vi "Sub_Saveas.vi"(7 "Template Name":string="saveas.xlsx", 8 "row":i32=2, 10 "File Name":refnum<vi>, 11 "Path":refnum<vi>) -> (3 "Save Path":path)   [LabVIEW 2015]
uses:
  buffer_mode.ctl
  <vilib>/Utility/NIReport.llb/NI_report.lvclass
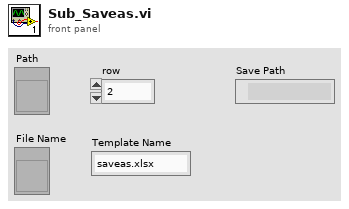
[diagram p1: front panel]
types:
  T1 = enum16{"maximized", "minimized", "normal", "no change"}
  T2 = enum16{"Standard Report", "HTML", "Word", "Excel"}
  T3 = typedef "buffer_mode.ctl" = enum16{"Clear", "Init", "Add 2nd data", "Delete", "Output"}
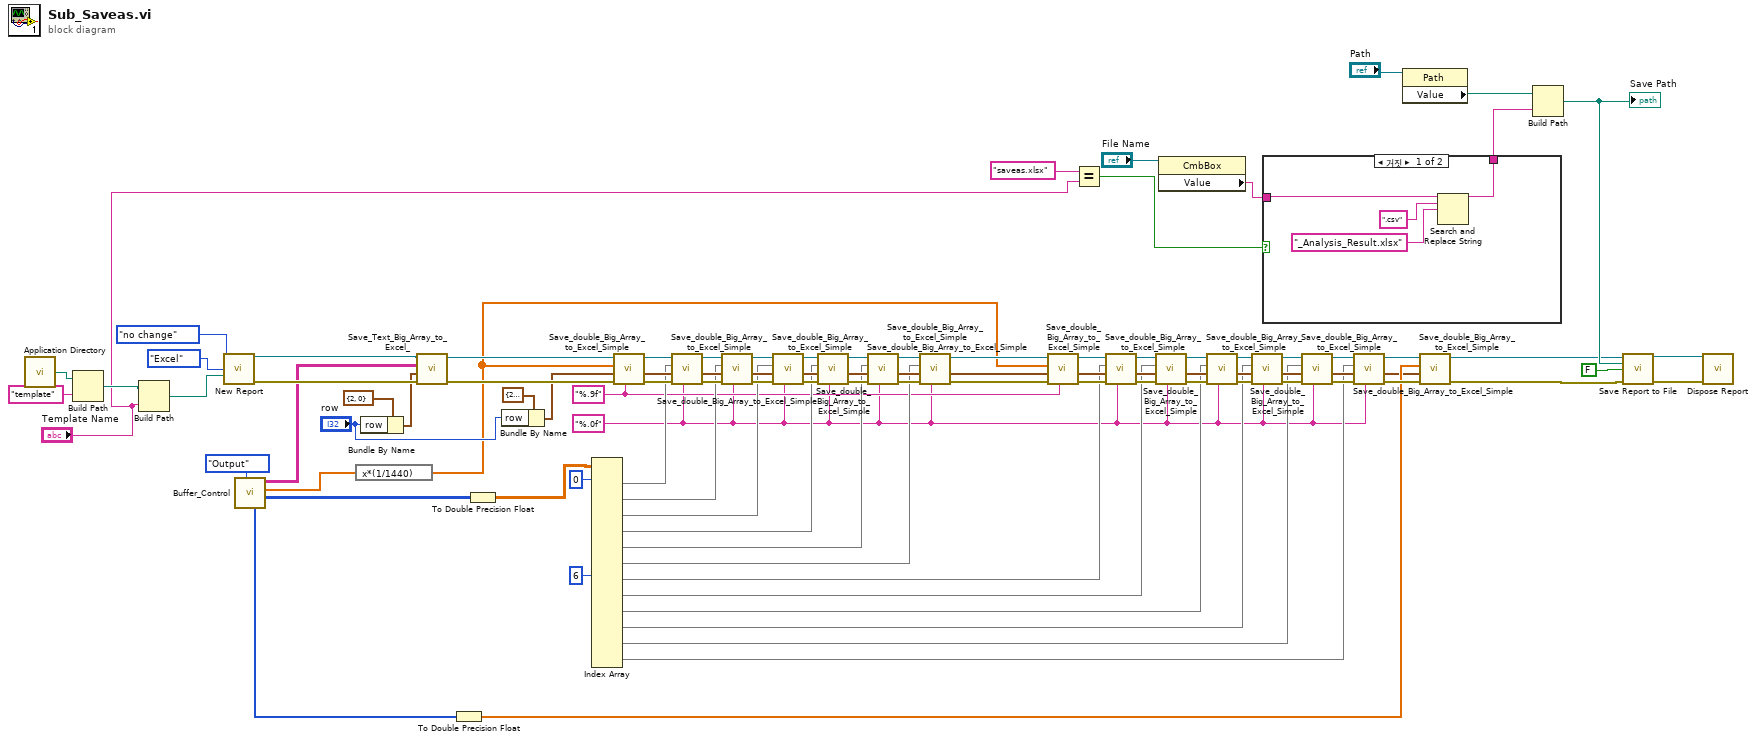
[diagram p0: block diagram]
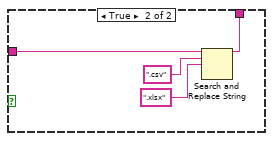
[diagram p2: hidden frame]
diagram:
  w18 = "%.0f" ("format string (%.3f)")
  w19 = "%.9f" ("format string (%.3f)")
  n1 = call <vilib>:"Application Directory.vi"() -> ("Application Directory"=w80:path)
  n2 = Build Path(base path=w80, name or relative path="template" ("이름 또는 상대 경로")) -> (appended path=w82:path)
  n3 = Build Path(base path=w82, name or relative path="Template Name") -> (appended path=w83:path)
  n4 = call <vilib>:"New Report.vi"("window state (normal)"=T1."no change", "report type"=T2."Excel", "template (empty)"=w83) -> ("report out"=w75:refnum<class "NI_report.lvclass">, "error out"=w73:errorcluster)  [unwired: 11 in]
  n5 = call "Buffer_Control.vi"("Mode"=buffer_mode."Output") -> ("Counts out"=w87:u32[][], "Timeline out"=w2:dbl[], "origin out"=w71:string[][], "Temp out"=w17:u32[])  [unwired: 6 in, 1 out]
  n6 = expression code="x*(1/1440)"(w2) -> (w1:dbl[])
  n7 = Bundle By Name(cluster=cluster{"row":i32, "column":i32} {"row"=2, "column"=0} ("start Position"), "row"="row") -> (w9:cluster{"row":i32, "column":i32})
  n8 = call "Save_Text_Big_Array_to_Excel_.vi"("error in (no error)"=w73, "start Position"=w9, "배열"=w71, "report in"=w75) -> ("error out"=w72:errorcluster, "report out"=w74:refnum<class "NI_report.lvclass">)  [unwired: 6 in]
  n9 = To Double Precision Float(number=w17) -> (double precision float=w14:dbl[])
  n10 = To Double Precision Float(number=w87) -> (double precision float=w88:dbl[][])
  n11 = Bundle By Name(cluster=cluster{"row":i32, "column":i32} {"row"=2, "column"=35} ("start (0, 0)"), "row"="row") -> (w6:cluster{"row":i32, "column":i32})
  n12 = Index Array(array=w88, index (row) #1=0 ("인덱스 (행)"), index (row) #7=6 ("인덱스 (행)")) -> (element #1=w67:dbl[], element #2=w60:dbl[], element #3=w59:dbl[], element #4=w55:dbl[], element #5=w51:dbl[], element #6=w47:dbl[], element #7=w25:dbl[], element #8=w24:dbl[], element #9=w23:dbl[], element #10=w22:dbl[], element #11=w21:dbl[], element #12=w20:dbl[])  [unwired: 22 in]
  n13 = call "Save_double_Big_Array_to_Excel_Simple.vi"("format string (%.3f)"=w19, "에러 입력(에러 없음)"=w72, "start (0, 0)"=w6, "배열"=w1, "NI_report 입력"=w74) -> ("error out"=w69:errorcluster, "Next Position"=w68:cluster{"row":i32, "column":i32}, "report out"=w70:refnum<class "NI_report.lvclass">)  [unwired: 4 in]
  n14 = call "Save_double_Big_Array_to_Excel_Simple.vi"("format string (%.3f)"=w18, "에러 입력(에러 없음)"=w69, "start (0, 0)"=w68, "배열"=w67, "NI_report 입력"=w70) -> ("error out"=w66:errorcluster, "Next Position"=w65:cluster{"row":i32, "column":i32}, "report out"=w64:refnum<class "NI_report.lvclass">)  [unwired: 4 in]
  n15 = call "Save_double_Big_Array_to_Excel_Simple.vi"("format string (%.3f)"=w18, "에러 입력(에러 없음)"=w66, "start (0, 0)"=w65, "배열"=w60, "NI_report 입력"=w64) -> ("error out"=w62:errorcluster, "Next Position"=w61:cluster{"row":i32, "column":i32}, "report out"=w63:refnum<class "NI_report.lvclass">)  [unwired: 4 in]
  n16 = call "Save_double_Big_Array_to_Excel_Simple.vi"("format string (%.3f)"=w18, "에러 입력(에러 없음)"=w62, "start (0, 0)"=w61, "배열"=w59, "NI_report 입력"=w63) -> ("error out"=w58:errorcluster, "Next Position"=w56:cluster{"row":i32, "column":i32}, "report out"=w57:refnum<class "NI_report.lvclass">)  [unwired: 4 in]
  n17 = call "Save_double_Big_Array_to_Excel_Simple.vi"("format string (%.3f)"=w18, "에러 입력(에러 없음)"=w58, "start (0, 0)"=w56, "배열"=w55, "NI_report 입력"=w57) -> ("error out"=w53:errorcluster, "Next Position"=w52:cluster{"row":i32, "column":i32}, "report out"=w54:refnum<class "NI_report.lvclass">)  [unwired: 4 in]
  n18 = call "Save_double_Big_Array_to_Excel_Simple.vi"("format string (%.3f)"=w18, "에러 입력(에러 없음)"=w53, "start (0, 0)"=w52, "배열"=w51, "NI_report 입력"=w54) -> ("error out"=w50:errorcluster, "Next Position"=w48:cluster{"row":i32, "column":i32}, "report out"=w49:refnum<class "NI_report.lvclass">)  [unwired: 4 in]
  n19 = call "Save_double_Big_Array_to_Excel_Simple.vi"("format string (%.3f)"=w18, "에러 입력(에러 없음)"=w50, "start (0, 0)"=w48, "배열"=w47, "NI_report 입력"=w49) -> ("error out"=w27:errorcluster, "Next Position"=w26:cluster{"row":i32, "column":i32}, "report out"=w28:refnum<class "NI_report.lvclass">)  [unwired: 4 in]
  n20 = call "Save_double_Big_Array_to_Excel_Simple.vi"("format string (%.3f)"=w19, "에러 입력(에러 없음)"=w27, "start (0, 0)"=w26, "배열"=w1, "NI_report 입력"=w28) -> ("error out"=w30:errorcluster, "Next Position"=w31:cluster{"row":i32, "column":i32}, "report out"=w29:refnum<class "NI_report.lvclass">)  [unwired: 4 in]
  n21 = Equal?(x="saveas.xlsx", y="Template Name") -> (x = y?=w4:bool)
  n22 = call "Save_double_Big_Array_to_Excel_Simple.vi"("format string (%.3f)"=w18, "에러 입력(에러 없음)"=w30, "start (0, 0)"=w31, "배열"=w25, "NI_report 입력"=w29) -> ("error out"=w32:errorcluster, "Next Position"=w33:cluster{"row":i32, "column":i32}, "report out"=w34:refnum<class "NI_report.lvclass">)  [unwired: 4 in]
  n23 = call "Save_double_Big_Array_to_Excel_Simple.vi"("format string (%.3f)"=w18, "에러 입력(에러 없음)"=w32, "start (0, 0)"=w33, "배열"=w24, "NI_report 입력"=w34) -> ("error out"=w36:errorcluster, "Next Position"=w37:cluster{"row":i32, "column":i32}, "report out"=w35:refnum<class "NI_report.lvclass">)  [unwired: 4 in]
  n24 = property class="CmbBox"(reference="File Name") -> ("Value"=w92:string)  [unwired: 1 in, 2 out]
  n25 = call "Save_double_Big_Array_to_Excel_Simple.vi"("format string (%.3f)"=w18, "에러 입력(에러 없음)"=w36, "start (0, 0)"=w37, "배열"=w23, "NI_report 입력"=w35) -> ("error out"=w38:errorcluster, "Next Position"=w40:cluster{"row":i32, "column":i32}, "report out"=w39:refnum<class "NI_report.lvclass">)  [unwired: 4 in]
  n26 = call "Save_double_Big_Array_to_Excel_Simple.vi"("format string (%.3f)"=w18, "에러 입력(에러 없음)"=w38, "start (0, 0)"=w40, "배열"=w22, "NI_report 입력"=w39) -> ("error out"=w42:errorcluster, "Next Position"=w43:cluster{"row":i32, "column":i32}, "report out"=w41:refnum<class "NI_report.lvclass">)  [unwired: 4 in]
  n27 = case shown="거짓" w4 {
    tunnel: [w96 w103] -> w93
    tunnel: w92 -> [w97 w100]
    frame False {
      n28 = Search and Replace String(input string=w97, search string=".csv" ("검색 문자열"), replace string="_Analysis_Result.xlsx" ("대체 문자열(\"\")")) -> (result string=w96:string)  [unwired: 5 in, 3 out]
    }
    frame True {
      n29 = Search and Replace String(input string=w100, search string=".csv" ("검색 문자열"), replace string=".xlsx" ("대체 문자열(\"\")")) -> (result string=w103:string)  [unwired: 5 in, 3 out]
    }
  }
  n30 = call "Save_double_Big_Array_to_Excel_Simple.vi"("format string (%.3f)"=w18, "에러 입력(에러 없음)"=w42, "start (0, 0)"=w43, "배열"=w21, "NI_report 입력"=w41) -> ("error out"=w44:errorcluster, "Next Position"=w46:cluster{"row":i32, "column":i32}, "report out"=w45:refnum<class "NI_report.lvclass">)  [unwired: 4 in]
  n31 = call "Save_double_Big_Array_to_Excel_Simple.vi"("format string (%.3f)"=w18, "에러 입력(에러 없음)"=w44, "start (0, 0)"=w46, "배열"=w20, "NI_report 입력"=w45) -> ("error out"=w16:errorcluster, "Next Position"=w13:cluster{"row":i32, "column":i32}, "report out"=w15:refnum<class "NI_report.lvclass">)  [unwired: 4 in]
  n32 = property class="Path"(reference="Path") -> ("Value"=w91:path)  [unwired: 1 in, 2 out]
  n33 = call "Save_double_Big_Array_to_Excel_Simple.vi"("에러 입력(에러 없음)"=w16, "start (0, 0)"=w13, "배열"=w14, "NI_report 입력"=w15) -> ("error out"=w11:errorcluster, "report out"=w12:refnum<class "NI_report.lvclass">)  [unwired: 5 in, 1 out]
  n34 = Build Path(base path=w91, name or relative path=w93) -> (appended path=w94:path)
  "Save Path" <- w94
  n35 = call-dynamic "Save Report to File.vi"("report in"=w12, "report file path"=w94, "prompt to replace? (F)"=FALSE, "error in (no error)"=w11) -> ("report out"=w89:refnum<class "NI_report.lvclass">, "error out"=w90:errorcluster)  [unwired: 10 in]
  n36 = call-dynamic "Dispose Report.vi"("report in"=w89, "error in (no error)"=w90) -> ()  [unwired: 13 in, 1 out]
